vi "Clear.vi"(8 "错误输入":errorcluster, 11 "Mlistbox Ref":refnum<vi>) -> (0 "错误输出":errorcluster, 3 "Mlistbox Ref Dup":refnum<vi>)   [LabVIEW 2012, in "Mlistbox Tools.lvlib"]
uses:
  Mlistbox Tools.lvlib
  ListBox/Custom Type/Read and Write Mode.ctl
  Property/Set and Get ItemNames.vi
  ListBox/Listbox Tool.lvlib
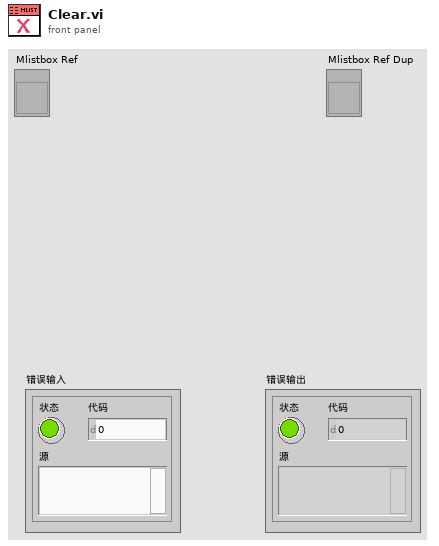
[diagram p1: front panel]
types:
  T1 = typedef "Listbox Tool.lvlib/Read and Write Mode.ctl" = enum16{"Read", "Write"}
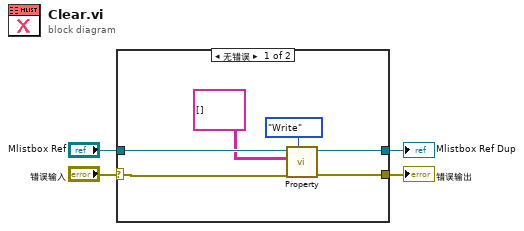
[diagram p0: block diagram]
diagram:
  n1 = case shown="无错误" "错误输入" {
    selector: "错误输入" -> [w5 w12]
    tunnel: [w8 w12] -> w3
    tunnel: "Mlistbox Ref" -> [w7 w11]
    tunnel: [w9 w11] -> w1
    frame No Error {
      n2 = call-poly "Property.vi"("Mode"=Read_and_Write_Mode."Write", "错误输入"=w5, "ItemNames In"=string[][] [], "Mlistbox Ref"=w7) -> ("错误输出"=w8:errorcluster, "Mlistbox Ref Dup"=w9:refnum<vi>)  [unwired: 5 in, 1 out]
    }
    frame Error {
    }
  }
  "Mlistbox Ref Dup" <- w1
  "错误输出" <- w3
